vi "Scintilla Move Scroll by Frame Num.vi"(8 "error in (no error)":errorcluster, 10 "Frame Number":u32, 11 "IDE simple in":refnum<class "Main Panel.lvclass">) -> (0 "error out":errorcluster, 3 "IDE simple out":refnum<class "Main Panel.lvclass">)   [LabVIEW 2018, in "Main Panel.lvlib" / "Main Panel.lvclass"]
uses:
  Main Panel.lvclass
  Main Panel.lvclass/Main Panel.ctl
  Frame Analizer/Data Parser.lvclass
  ScintillaNET/ScintillaNET.lvclass
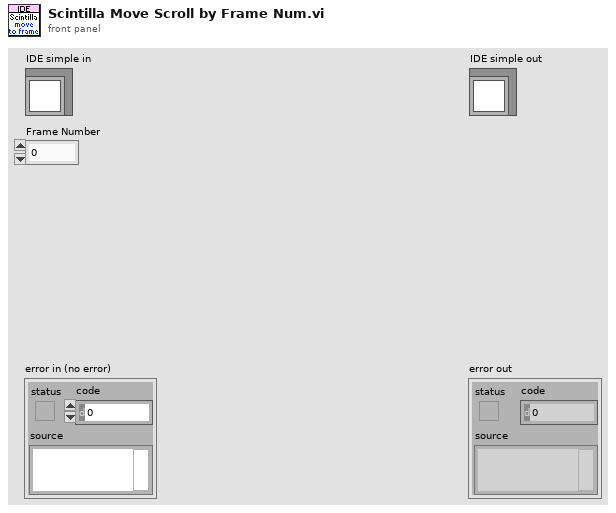
[diagram p1: front panel]
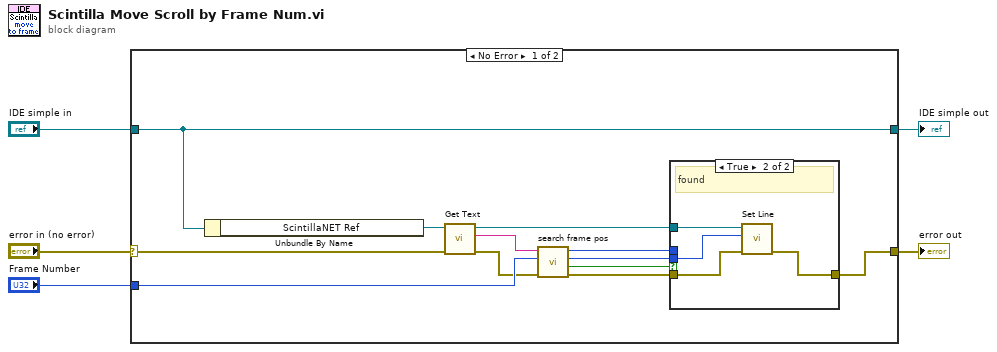
[diagram p0: block diagram]
diagram:
  n1 = case shown="No Error" "error in (no error)" {
    selector: "error in (no error)" -> [w9 w24]
    tunnel: [w13 w24] -> w4
    tunnel: [w7 w23] -> w2
    tunnel: "IDE simple in" -> [w7 w23]
    tunnel: "Frame Number" -> [w17 _]
    frame No Error {
      n2 = Unbundle By Name(w7) -> ("ScintillaNET Ref"=w10:refnum<class "ScintillaNET.lvclass">)
      n3 = call "Get Text.vi"("error in (no error)"=w9, "ScintillaNET in"=w10) -> ("error out"=w6:errorcluster, "Text"=w11:string, "ScintillaNET out"=w8:refnum<class "ScintillaNET.lvclass">)  [unwired: 7 in]
      n4 = call "search frame pos.vi"("error in (no error)"=w6, "Frame Number"=w17, "String"=w11) -> ("error out"=w14:errorcluster, "Found"=w12:bool, "Line Num"=w16:i32, "Position"=w15:i32)  [unwired: 5 in]
      n5 = case shown="True" w12 {
        tunnel: w16 -> [_ w21]
        tunnel: w15 -> [_ _]
        tunnel: w14 -> [w18 w20]
        tunnel: [w18 w19] -> w13
        tunnel: w8 -> [_ w22]
        frame False {
          # "not found"
        }
        frame True {
          # "found"
          n6 = call "Set Line.vi"("error in (no error)"=w20, "First Visible Line"=w21, "ScintillaNET in"=w22) -> ("error out"=w19:errorcluster)  [unwired: 7 in, 1 out]
        }
      }
    }
    frame Error {
    }
  }
  "error out" <- w4
  "IDE simple out" <- w2
